vi "run script line.vi"(8 "error in (no error)":errorcluster caption="에러 입력(에러 없음)", 11 "Script Line_i2c w 입력":refnum<class "Script Line_i2c w.lvclass">) -> (0 "error out":errorcluster caption="에러 출력", 2 "log":string, 3 "Script Line_i2c w 출력":refnum<class "Script Line_i2c w.lvclass">)   [LabVIEW 2020, in "Script Line_i2c w.lvclass"]
uses:
  Script Line_i2c w.lvclass
  Script Line_i2c/Script Line_i2c.lvclass/Script Line_i2c.ctl
  Script Line_i2c/Accessors/Read reg.vi
  Script Line_i2c/Accessors/Read data.vi
  Script Line_i2c/Accessors/Read slv.vi
  Script Line_i2c/Accessors/Read reg addr byte.vi
  BD Protocol Class/I2C/I2C.lvclass
  Script Line_i2c/Script Line_i2c.lvclass
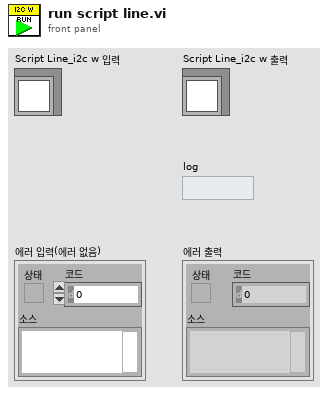
[diagram p1: front panel]
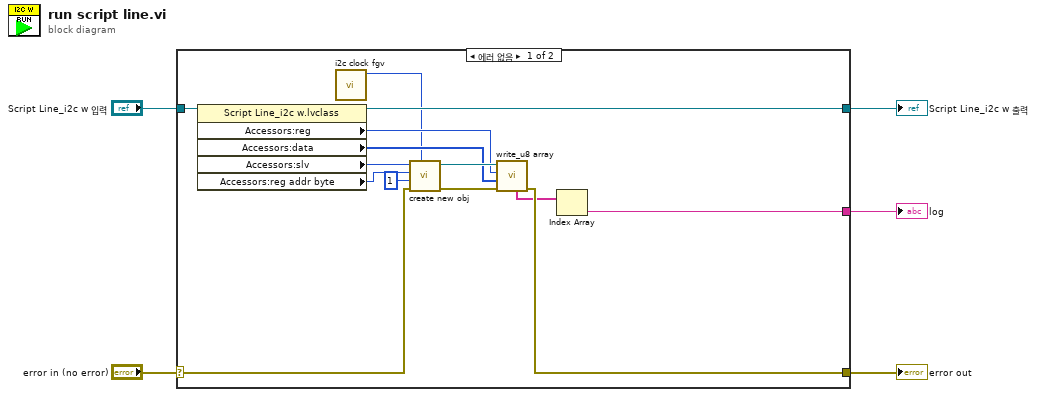
[diagram p0: block diagram]
diagram:
  n1 = case shown="에러 없음" "error in (no error)" {
    selector: "error in (no error)" -> [w16 w21]
    tunnel: [w15 w21] -> w5
    tunnel: [w9 w20] -> w4
    tunnel: "Script Line_i2c w 입력" -> [w14 w20]
    tunnel: [w8 _] -> w1
    frame No Error {
      n2 = property class="Script Line_i2c w.lvclass"(reference=w14) -> (reference out=w9:refnum<class "Script Line_i2c w.lvclass">, "Accessors:reg"=w13:u32, "Accessors:data"=w12:u8[], "Accessors:slv"=w11:u8, "Accessors:reg addr byte"=w10:u8)  [unwired: 1 in, 1 out]
      n3 = call "i2c clock fgv.vi"() -> ("i2c clock out"=w7:u8)  [unwired: 10 in, 1 out]
      n4 = call "create new obj.vi"("clock rate"=w7, "error in (no error)"=w16, "data byte"=u8 1 ("address byte"), "address byte"=w10, "slave address"=w11) -> ("error out"=w17:errorcluster, "new I2C obj"=w18:refnum<class "I2C.lvclass">)  [unwired: 5 in]
      n5 = call-dynamic "write_u8 array.vi"("error in (no error)"=w17, "data to write"=w12, "start address"=w13, "I2C 입력"=w18) -> ("error out"=w15:errorcluster, "log_single line"=w6:string[])  [unwired: 3 in, 3 out]
      n6 = Index Array(array=w6) -> (element=w8:string)  [unwired: 1 in]
    }
    frame Error {
    }
  }
  "error out" <- w5
  "Script Line_i2c w 출력" <- w4
  "log" <- w1
